vi "Themocouple Test2.vi"() -> ()   [LabVIEW 2018]
uses:
  <vilib>/DAQmx/read.llb/DAQmx Read.vi
  <vilib>/DAQmx/read.llb/DAQmx Read (Analog 1D Wfm NChan NSamp).vi
  <vilib>/DAQmx/miscellaneous.llb/DAQmx Fill In Error Info.vi
panel:
  out "data":waveform(dbl)[](graph)
  in  "stop":bool
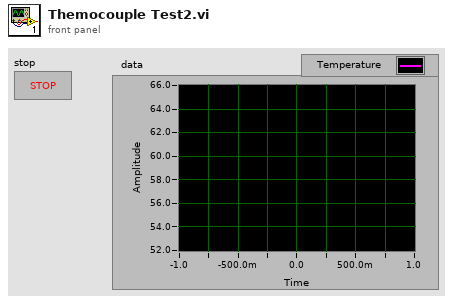
[diagram p1: front panel]
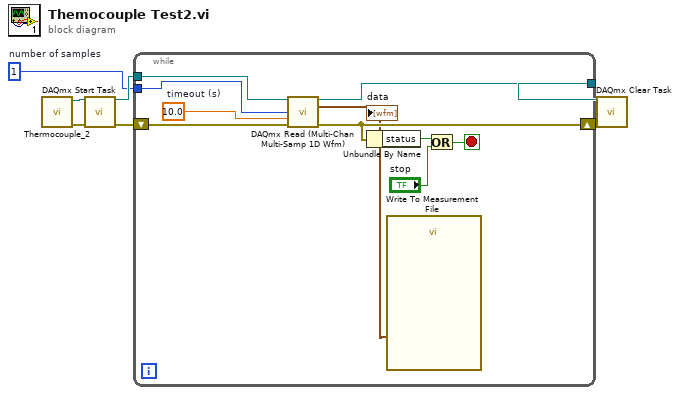
[diagram p0: block diagram]
diagram:
  w5 = 1  # number of samples
  n1 = call "Thermocouple_2.vi"() -> ("error out"=w1:errorcluster, "task out"=w2:refnum<k21>)  [unwired: 10 in]
  n2 = call <vilib>:"DAQmx Start Task.vi"("task/channels in"=w2, "error in"=w1) -> ("task out"=w7:refnum<k21>, "error out"=w6:errorcluster)  [unwired: 12 in]
  n3 = while {
    tunnel: w7 -> [w17]
    tunnel: w5 -> [w14]
    tunnel: [w15] -> w3
    shift-right: [w12] -> w4
    shift-left: w6 -> [w16]
    stop <- w11 stop-if-true
    w9 = 10.0  # timeout (s)
    n4 = call-poly "DAQmx Read (Multi-Chan Multi-Samp 1D Wfm).vi"("task/channels in"=w17, "number of samples per channel"=w14, "timeout"=w9, "error in"=w16) -> ("task out"=w15:refnum<k21>, "data"=w8:waveform(dbl)[], "error out"=w12:errorcluster)  [unwired: 9 in]
    "data" <- w8
    n5 = Unbundle By Name(w12) -> ("status"=w13:bool)
    n6 = call "Write To Measurement File"("Signals"=w8) -> ()  [unwired: 16 in, 3 out]
    n7 = Or(x=w13, y="stop") -> (x .or. y?=w11:bool)
  }
  n8 = call <vilib>:"DAQmx Clear Task.vi"("task in"=w3, "error in"=w4) -> ()  [unwired: 13 in, 1 out]
